vi "array - generate arctan range.vi.vi"(6 "N":i32=-1, 10 "omega0":dbl, 11 "gamma":dbl) -> (0 "Array":dbl[](array[numeric]))   [LabVIEW 2018]
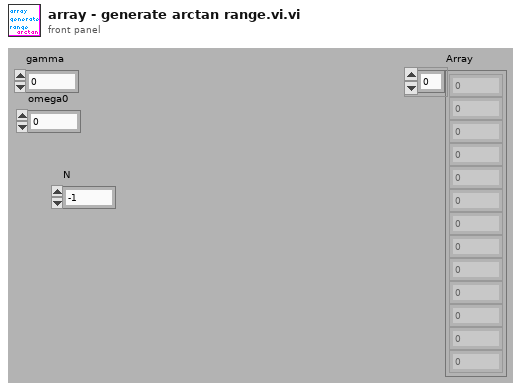
[diagram p1: front panel]
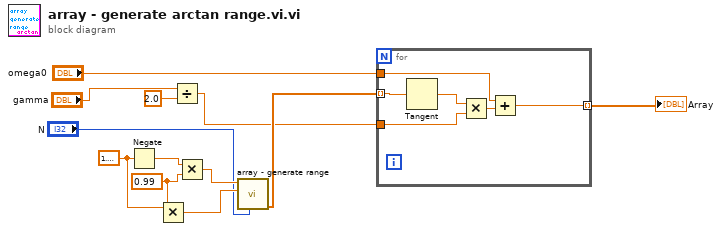
[diagram p0: block diagram]
diagram:
  w9 = 0.99
  w10 = 1.5707963267948966
  n1 = Negate(x=w10) -> (-x=w11:dbl)
  n2 = Multiply(x=w10, y=w9) -> (x*y=w7:dbl)
  n3 = Divide(x="gamma", y=2.0) -> (x/y=w1:dbl)
  n4 = Multiply(x=w11, y=w9) -> (x*y=w8:dbl)
  n5 = call "array - generate range.vi"("N"="N", "freq max"=w7, "freq min"=w8) -> ("Array"=w5:dbl[])  [unwired: 7 in, 1 out]
  n6 = for {
    tunnel: [w18] -> w12 mode=indexing
    tunnel: w5 -> [w16] mode=indexing
    tunnel: "omega0" -> [w17]
    tunnel: w1 -> [w15]
    n7 = Tangent(1:w16) -> (0:w14:dbl)
    n8 = Multiply(x=w14, y=w15) -> (x*y=w13:dbl)
    n9 = Add(x=w17, y=w13) -> (x+y=w18:dbl)
  }
  "Array" <- w12
